vi "Kinesis-Teste-Vector-3.vi"() -> ()   [LabVIEW 2014]
doc: "André Romero - 2017\nandretec@ifsc.usp.br"
uses:
  Basic-VIs/motorsGlobalVar.vi
  <vilib>/Instr/_visa.llb/VISA Configure Serial Port (Instr).vi
  C:/user-Lab/AndreTec/GITs/andretec/Thorlabs-Vector-Move/kinesisTec/Kinesis/Thorlabs.MotionControl.Controls.dll
  kinesisTec/Kinesis/Thorlabs.MotionControl.Controls.dll
panel:
  out "IsMoving Y":bool
  out "IsMoving X":bool
  out "Y":dbl[](array[numeric])
  out "X":dbl[](array[numeric])
  out "XY Graph 2":cluster{dbl[], dbl[]}(graph)={[0.0, 0.8660254037844387, -0.8660254037844384, 0.0], [1.0, -0.4999999999999998, -0.5000000000000004, 1.0]}
  in  "Adjust Motors":bool
  out "Process time":string="0:00:50"
  out "Progress %":dbl(slide) scale=0.0..100.0
  out "XY Graph":cluster{"Graph X":dbl[], "Graph Y":dbl[]}(graph)
  in  "Swap XY":bool
  out "stop cronometro":bool=TRUE
  in  "Stop Button":bool
  in  "Graph Y":dbl[](array[numeric])=[0.0, 0.0, 6.6674440298507465, 6.6674440298507465, 6.6674440298507465, 6.6674440298507465, 6.6674440298507465, 6.6674440298507465, 6.6674440298507465, 6.6674440298507465, 6.6674440298507465, 6.6674440298507465, 6.6674440298507465, 6.6674440298507465, 6.6674440298507465, 6.6674440298507465, 6.6674440298507465, 6.6674440298507465, 6.6674440298507465, 6.6674440298507465, 6.6674440298507465, 6.6674440298507465, 6.6674440298507465, 6.6674440298507465, 6.6674440298507465, 6.6674440298507465, 6.6674440298507465, 6.6674440298507465, 6.6674440298507465, 6.6674440298507465, 6.6674440298507465, 6.6674440298507465, 6.6674440298507465, 6.6674440298507465, 6.6674440298507465, 6.6674440298507465, 6.6674440298507465, 6.6674440298507465, 6.6674440298507465, 6.6674440298507465, 6.6674440298507465, 6.6674440298507465, 6.6674440298507465, 6.673128498134329, 6.673128498134329, 6.673128498134329, 6.673128498134329, 6.673128498134329, 6.687354244402985, 6.687354244402985, 6.687354244402985, 6.687354244402985, 6.687354244402985, 6.692543143656716, 6.692543143656716, 6.692543143656716, 6.692543143656716, 6.692543143656716, 6.692543143656716, 6.692543143656716, 6.692543143656716, 6.692543143656716, 6.692543143656716, 6.692543143656716, 6.692543143656716, 6.691522854477612, 6.691522854477612, 6.691522854477612, 6.691522854477612, 6.691522854477612, 6.680183069029851, 6.680183069029851, 6.680183069029851, 6.680183069029851, 6.680183069029851, 6.658640391791045, 6.658640391791045, 6.658640391791045, 6.658640391791045, 6.658640391791045, 6.644793610074627, 6.644793610074627, 6.644793610074627, 6.644793610074627, 6.644793610074627, 6.642490671641791, 6.642490671641791, 6.642490671641791, 6.642490671641791, 6.642490671641791, 6.642490671641791, 6.642490671641791, 6.642490671641791, 6.642490671641791, 6.642490671641791, 6.642490671641791, 6.642490671641791, 6.642490671641791, 6.642490671641791, 6.642490671641791, 6.647825326492537, 6.647825326492537, 6.647825326492537, 6.647825326492537, 6.647825326492537, 6.66543260261194, 6.66543260261194, 6.66543260261194, 6.66543260261194, 6.66543260261194, 6.685226212686567, 6.685226212686567, 6.685226212686567, 6.685226212686567, 6.685226212686567, 6.692484841417911, 6.692484841417911, 6.692484841417911, 6.692484841417911, 6.692484841417911, 6.692543143656716, 6.692543143656716, 6.692543143656716, 6.692543143656716, 6.692543143656716, 6.692543143656716, 6.692543143656716, 6.691464552238806, 6.691464552238806, 6.691464552238806, 6.691464552238806, 6.691464552238806, 6.679833255597015, 6.679833255597015, 6.679833255597015, 6.679833255597015, 6.679833255597015, 6.658057369402985, 6.658057369402985, 6.658057369402985, 6.658057369402985, 6.658057369402985, 6.644647854477612, 6.644647854477612, 6.644647854477612, 6.644647854477612, 6.644647854477612, 6.642548973880597, 6.642548973880597, 6.642548973880597, 6.642548973880597, 6.642548973880597, 6.642519822761194, 6.642519822761194, 6.642519822761194, 6.642519822761194, 6.642519822761194, 6.642519822761194, 6.642519822761194, 6.642519822761194, 6.643569263059701, 6.643569263059701, 6.643569263059701, 6.643569263059701, 6.643569263059701, 6.655521222014926, 6.655521222014926, 6.655521222014926, 6.655521222014926, 6.655521222014926, 6.677180503731344, 6.677180503731344, 6.677180503731344, 6.677180503731344, 6.677180503731344, 6.690531716417911, 6.690531716417911, 6.690531716417911, 6.690531716417911, 6.690531716417911, 6.692572294776119, 6.692572294776119, 6.692572294776119, 6.692572294776119, 6.692572294776119, 6.692572294776119, 6.692572294776119, 6.692572294776119, 6.692572294776119, 6.692572294776119, 6.692572294776119, 6.692572294776119, 6.691522854477612, 6.691522854477612, 6.691522854477612, 6.691522854477612, 6.691522854477612, 6.680008162313433, 6.680008162313433, 6.680008162313433, 6.680008162313433, 6.680008162313433, 6.668668376865671, 6.668668376865671, 6.668668376865671, 6.668668376865671, 6.668668376865671, 6.667502332089552, 6.667502332089552, 6.667502332089552, 6.667502332089552, 6.667502332089552, 6.667502332089552, 6.667502332089552, 6.667502332089552, 6.667502332089552, 6.667502332089552, 6.667502332089552, 6.667502332089552, 6.667531483208955, 6.667531483208955, 6.667531483208955, 6.667531483208955, 6.667531483208955, 6.667531483208955, 6.667531483208955, 6.667531483208955, 6.667531483208955, 6.667531483208955, 6.667531483208955, 6.667531483208955, 6.667531483208955, 6.667531483208955, 6.667531483208955, 6.667531483208955, 6.667531483208955, 6.667531483208955, 6.667531483208955, 6.667531483208955, 6.667531483208955, 6.667531483208955, 6.667531483208955, 6.667531483208955, 6.667531483208955, 6.667531483208955, 6.667531483208955, 6.667531483208955, 6.667531483208955, 6.667531483208955, 6.667531483208955, 6.667531483208955, 6.667531483208955, 6.667531483208955, 6.667531483208955, 6.667531483208955, 6.667531483208955, 6.6663945895522385, 6.6663945895522385, 6.6663945895522385, 6.6663945895522385, 6.6663945895522385, 6.662051072761194, 6.662051072761194, 6.662051072761194, 6.662051072761194, 6.662051072761194, 6.644035680970149, 6.644035680970149, 6.644035680970149, 6.644035680970149, 6.644035680970149, 6.606430736940299, 6.606430736940299, 6.606430736940299, 6.606430736940299, 6.606430736940299, 6.593924906716418, 6.593924906716418, 6.593924906716418, 6.593924906716418, 6.593924906716418, 6.574539412313433, 6.574539412313433, 6.574539412313433, 6.574539412313433, 6.574539412313433, 6.567484841417911, 6.567484841417911, 6.567484841417911, 6.567484841417911, 6.567484841417911, 6.567484841417911, 6.567484841417911, 6.567484841417911, 6.567484841417911, 6.567484841417911, 6.567484841417911, 6.567513992537314, 6.567513992537314, 6.567513992537314, 6.567513992537314, 6.567513992537314, 6.567513992537314, 6.567513992537314, 6.567513992537314, 6.567513992537314, 6.567513992537314, 6.567543143656716, 6.567543143656716, 6.567543143656716, 6.567543143656716, 6.567543143656716, 6.567543143656716, 6.567543143656716, 6.567543143656716, 6.567543143656716, 6.567543143656716, 6.567543143656716, 6.567543143656716, 6.567543143656716, 6.567543143656716, 6.567543143656716, 6.567543143656716, 6.567543143656716, 6.567543143656716, 6.567543143656716, 6.567543143656716, 6.567543143656716, 6.567543143656716, 6.567543143656716, 6.567543143656716, 6.567543143656716, 6.567543143656716, 6.567543143656716, 6.567543143656716, 6.567543143656716, 6.567543143656716, 6.567543143656716, 6.567543143656716, 6.567543143656716, 6.567543143656716, 6.567543143656716, 6.567543143656716, 6.567543143656716, 6.567543143656716, 6.567543143656716, 6.567543143656716, 6.567543143656716, 6.567543143656716, 6.567543143656716, 6.567543143656716, 6.567543143656716, 6.567543143656716, 6.567543143656716, 6.567543143656716, 6.567543143656716, 6.567543143656716, 6.567543143656716, 6.567543143656716, 6.567543143656716, 6.567543143656716, 6.5667852145522385, 6.5667852145522385, 6.5667852145522385, 6.5667852145522385, 6.5667852145522385, 6.555299673507463, 6.555299673507463, 6.555299673507463, 6.555299673507463, 6.555299673507463, 6.533523787313433, 6.533523787313433, 6.533523787313433, 6.533523787313433, 6.533523787313433, 6.525186567164179, 6.525186567164179, 6.525186567164179, 6.525186567164179, 6.525186567164179, 6.517490671641791, 6.517490671641791, 6.517490671641791, 6.517490671641791, 6.517490671641791, 6.517490671641791, 6.517490671641791, 6.517490671641791, 6.517490671641791, 6.517490671641791, 6.517519822761194, 6.517519822761194, 6.517519822761194, 6.517519822761194, 6.517519822761194, 6.517519822761194, 6.517519822761194, 6.517519822761194, 6.517519822761194, 6.517519822761194, 6.517548973880597, 6.517548973880597, 6.517548973880597, 6.517548973880597, 6.517548973880597, 6.517548973880597, 6.517548973880597, 6.517548973880597, 6.517548973880597, 6.517548973880597, 6.517548973880597, 6.517548973880597, 6.517548973880597, 6.517548973880597, 6.517548973880597, 6.517548973880597, 6.517548973880597, 6.517548973880597, 6.517548973880597, 6.517548973880597, 6.517548973880597, 6.517548973880597, 6.517548973880597, 6.517548973880597, 6.517548973880597, 6.517548973880597, 6.517548973880597, 6.517548973880597, 6.517548973880597, 6.517548973880597, 6.517548973880597, 6.517548973880597, 6.517548973880597, 6.517548973880597, 6.517548973880597, 6.517548973880597, 6.517548973880597, 6.517548973880597, 6.517548973880597, 6.517548973880597, 6.517548973880597, 6.517548973880597, 6.517548973880597, 6.517548973880597, 6.517548973880597, 6.517548973880597, 6.517548973880597, 6.517548973880597, 6.517548973880597, 6.517548973880597, 6.517548973880597, 6.517548973880597, 6.517548973880597, 6.517548973880597, 6.517548973880597, 6.517548973880597, 6.517548973880597, 6.517548973880597, 6.517548973880597, 6.517548973880597, 6.516674440298507, 6.516674440298507, 6.516674440298507, 6.516674440298507, 6.516674440298507, 6.504897388059701, 6.504897388059701, 6.504897388059701, 6.504897388059701, 6.504897388059701, 6.481926305970149, 6.481926305970149, 6.481926305970149, 6.481926305970149, 6.481926305970149, 6.456943796641791, 6.456943796641791, 6.456943796641791, 6.456943796641791, 6.456943796641791, 6.4330690298507465, 6.4330690298507465, 6.4330690298507465, 6.4330690298507465, 6.4330690298507465, 6.419717817164179, 6.419717817164179, 6.419717817164179, 6.419717817164179, 6.419717817164179, 6.417473180970149, 6.417473180970149, 6.417473180970149, 6.417473180970149, 6.417473180970149, 6.417473180970149]
  in  "Graph X":dbl[](array[numeric])=[0.0, 0.0, 3.605935167910448, 3.605935167910448, 3.605935167910448, 3.605935167910448, 3.605935167910448, 3.609987173507463, 3.609987173507463, 3.609987173507463, 3.609987173507463, 3.609987173507463, 3.627157182835821, 3.627157182835821, 3.627157182835821, 3.627157182835821, 3.627157182835821, 3.6520813899253732, 3.6520813899253732, 3.6520813899253732, 3.6520813899253732, 3.6520813899253732, 3.6770930503731343, 3.6770930503731343, 3.6770930503731343, 3.6770930503731343, 3.6770930503731343, 3.697323927238806, 3.697323927238806, 3.697323927238806, 3.697323927238806, 3.697323927238806, 3.705311333955224, 3.705311333955224, 3.705311333955224, 3.705311333955224, 3.705311333955224, 3.705311333955224, 3.705311333955224, 3.705311333955224, 3.705311333955224, 3.705311333955224, 3.705311333955224, 3.7063024720149254, 3.7063024720149254, 3.7063024720149254, 3.7063024720149254, 3.7063024720149254, 3.7175839552238807, 3.7175839552238807, 3.7175839552238807, 3.7175839552238807, 3.7175839552238807, 3.7291861007462686, 3.7291861007462686, 3.7291861007462686, 3.7291861007462686, 3.7291861007462686, 3.7303521455223883, 3.7303521455223883, 3.7303521455223883, 3.7303521455223883, 3.7303521455223883, 3.7303521455223883, 3.7303521455223883, 3.7303521455223883, 3.7303521455223883, 3.7303521455223883, 3.7303521455223883, 3.7303521455223883, 3.7366779384328357, 3.7366779384328357, 3.7366779384328357, 3.7366779384328357, 3.7366779384328357, 3.7554221082089554, 3.7554221082089554, 3.7554221082089554, 3.7554221082089554, 3.7554221082089554, 3.774137126865672, 3.774137126865672, 3.774137126865672, 3.774137126865672, 3.774137126865672, 3.7803463152985075, 3.7803463152985075, 3.7803463152985075, 3.7803463152985075, 3.7803463152985075, 3.7803463152985075, 3.7803463152985075, 3.7803463152985075, 3.7803463152985075, 3.7803463152985075, 3.7803463152985075, 3.7803463152985075, 3.7803463152985075, 3.7803463152985075, 3.7803463152985075, 3.781803871268657, 3.781803871268657, 3.781803871268657, 3.781803871268657, 3.781803871268657, 3.7941930970149254, 3.7941930970149254, 3.7941930970149254, 3.7941930970149254, 3.7941930970149254, 3.816027285447761, 3.816027285447761, 3.816027285447761, 3.816027285447761, 3.816027285447761, 3.828678871268657, 3.828678871268657, 3.828678871268657, 3.828678871268657, 3.828678871268657, 3.8303404850746268, 3.8303404850746268, 3.8303404850746268, 3.8303404850746268, 3.8303404850746268, 3.8303404850746268, 3.8303404850746268, 3.8303404850746268, 3.8303404850746268, 3.8303404850746268, 3.8303404850746268, 3.8303404850746268, 3.8368703358208953, 3.8368703358208953, 3.8368703358208953, 3.8368703358208953, 3.8368703358208953, 3.8447994402985075, 3.8447994402985075, 3.8447994402985075, 3.8447994402985075, 3.8447994402985075, 3.866633628731343, 3.866633628731343, 3.866633628731343, 3.866633628731343, 3.866633628731343, 3.8803346548507465, 3.8803346548507465, 3.8803346548507465, 3.8803346548507465, 3.8803346548507465, 3.8803346548507465, 3.8803346548507465, 3.8803346548507465, 3.8803346548507465, 3.8803346548507465, 3.8803346548507465, 3.8803346548507465, 3.8803346548507465, 3.8803346548507465, 3.8803346548507465, 3.8803346548507465, 3.8803346548507465, 3.8803346548507465, 3.886631296641791, 3.886631296641791, 3.886631296641791, 3.886631296641791, 3.886631296641791, 3.9054046175373136, 3.9054046175373136, 3.9054046175373136, 3.9054046175373136, 3.9054046175373136, 3.92411963619403, 3.92411963619403, 3.92411963619403, 3.92411963619403, 3.92411963619403, 3.9303288246268657, 3.9303288246268657, 3.9303288246268657, 3.9303288246268657, 3.9303288246268657, 3.9303288246268657, 3.9303288246268657, 3.9303288246268657, 3.9303288246268657, 3.9303288246268657, 3.9303288246268657, 3.9303288246268657, 3.9303288246268657, 3.9303288246268657, 3.9303288246268657, 3.9303288246268657, 3.9303288246268657, 3.936800373134328, 3.936800373134328, 3.936800373134328, 3.936800373134328, 3.936800373134328, 3.9445545708955225, 3.9445545708955225, 3.9445545708955225, 3.9445545708955225, 3.9445545708955225, 3.95536963619403, 3.95536963619403, 3.95536963619403, 3.95536963619403, 3.95536963619403, 3.95536963619403, 3.95536963619403, 3.95536963619403, 3.95536963619403, 3.95536963619403, 3.95536963619403, 3.95536963619403, 3.956652285447761, 3.956652285447761, 3.956652285447761, 3.956652285447761, 3.956652285447761, 3.961141557835821, 3.961141557835821, 3.961141557835821, 3.961141557835821, 3.961141557835821, 3.9795067630597014, 3.9795067630597014, 3.9795067630597014, 3.9795067630597014, 3.9795067630597014, 4.004518423507463, 4.004518423507463, 4.004518423507463, 4.004518423507463, 4.004518423507463, 4.0406366604477615, 4.0406366604477615, 4.0406366604477615, 4.0406366604477615, 4.0406366604477615, 4.048624067164179, 4.048624067164179, 4.048624067164179, 4.048624067164179, 4.048624067164179, 4.0553579757462686, 4.0553579757462686, 4.0553579757462686, 4.0553579757462686, 4.0553579757462686, 4.0553579757462686, 4.0553579757462686, 4.055387126865671, 4.055387126865671, 4.055387126865671, 4.055387126865671, 4.055387126865671, 4.055387126865671, 4.055387126865671, 4.055387126865671, 4.055387126865671, 4.055387126865671, 4.0553579757462686, 4.0553579757462686, 4.0553579757462686, 4.0553579757462686, 4.0553579757462686, 4.0553579757462686, 4.0553579757462686, 4.0553579757462686, 4.0553579757462686, 4.0553579757462686, 4.0553579757462686, 4.0553579757462686, 4.0553579757462686, 4.0553579757462686, 4.0553579757462686, 4.0553579757462686, 4.0553579757462686, 4.0553579757462686, 4.0553579757462686, 4.0553579757462686, 4.0553579757462686, 4.0553579757462686, 4.0553579757462686, 4.0553579757462686, 4.0553579757462686, 4.0553579757462686, 4.0553579757462686, 4.0553579757462686, 4.0553579757462686, 4.0553579757462686, 4.0553579757462686, 4.061800373134329, 4.061800373134329, 4.061800373134329, 4.061800373134329, 4.061800373134329, 4.06972947761194, 4.06972947761194, 4.06972947761194, 4.06972947761194, 4.06972947761194, 4.091534514925373, 4.091534514925373, 4.091534514925373, 4.091534514925373, 4.091534514925373, 4.105352145522388, 4.105352145522388, 4.105352145522388, 4.105352145522388, 4.105352145522388, 4.105381296641791, 4.105381296641791, 4.105381296641791, 4.105381296641791, 4.105381296641791, 4.105381296641791, 4.105381296641791, 4.1050897854477615, 4.1050897854477615, 4.1050897854477615, 4.1050897854477615, 4.1050897854477615, 4.0951784048507465, 4.0951784048507465, 4.0951784048507465, 4.0951784048507465, 4.0951784048507465, 4.073489972014926, 4.073489972014926, 4.073489972014926, 4.073489972014926, 4.073489972014926, 4.060954990671642, 4.060954990671642, 4.060954990671642, 4.060954990671642, 4.060954990671642, 4.023874766791045, 4.023874766791045, 4.023874766791045, 4.023874766791045, 4.023874766791045, 4.008687033582089, 4.008687033582089, 4.008687033582089, 4.008687033582089, 4.008687033582089, 4.005363805970149, 4.005363805970149, 4.005363805970149, 4.005363805970149, 4.005363805970149, 4.005363805970149, 4.005363805970149, 4.005363805970149, 4.005363805970149, 4.005363805970149, 4.005363805970149, 4.005363805970149, 4.005363805970149, 4.005363805970149, 4.005363805970149, 4.005363805970149, 4.005363805970149, 4.005392957089552, 4.005392957089552, 4.005392957089552, 4.005392957089552, 4.005392957089552, 4.005392957089552, 4.005392957089552, 4.005392957089552, 4.005392957089552, 4.005392957089552, 4.005392957089552, 4.005392957089552, 4.005392957089552, 4.005392957089552, 4.005392957089552, 4.005392957089552, 4.005392957089552, 4.005392957089552, 4.005392957089552, 4.005392957089552, 4.011631296641791, 4.011631296641791, 4.011631296641791, 4.011631296641791, 4.011631296641791, 4.019472947761194, 4.019472947761194, 4.019472947761194, 4.019472947761194, 4.019472947761194, 4.042852145522388, 4.042852145522388, 4.042852145522388, 4.042852145522388, 4.042852145522388, 4.080398787313433, 4.080398787313433, 4.080398787313433, 4.080398787313433, 4.080398787313433, 4.099113805970149, 4.099113805970149, 4.099113805970149, 4.099113805970149, 4.099113805970149, 4.103777985074627, 4.103777985074627, 4.103777985074627, 4.103777985074627, 4.103777985074627, 4.105410447761194, 4.105410447761194, 4.105410447761194, 4.105410447761194, 4.105410447761194, 4.105410447761194, 4.105410447761194, 4.105410447761194, 4.105381296641791, 4.105381296641791, 4.105381296641791, 4.105381296641791, 4.105381296641791, 4.098297574626866, 4.098297574626866, 4.098297574626866, 4.098297574626866, 4.098297574626866, 4.089989505597015, 4.089989505597015, 4.089989505597015, 4.089989505597015, 4.089989505597015, 4.06083838619403, 4.06083838619403, 4.06083838619403, 4.06083838619403, 4.06083838619403, 4.0553579757462686, 4.0553579757462686, 4.0553579757462686, 4.0553579757462686, 4.0553579757462686, 4.0553579757462686, 4.0553579757462686, 4.0553579757462686, 4.0553579757462686, 4.0553579757462686, 4.0553579757462686, 4.0553579757462686, 4.055387126865671, 4.055387126865671, 4.055387126865671, 4.055387126865671, 4.055387126865671, 4.055416277985074, 4.055416277985074, 4.055416277985074, 4.055416277985074, 4.055416277985074, 4.055416277985074, 4.055416277985074, 4.055416277985074, 4.055416277985074, 4.055416277985074, 4.055416277985074, 4.055416277985074, 4.055416277985074, 4.055416277985074, 4.055416277985074, 4.055416277985074, 4.055416277985074, 4.055416277985074, 4.055416277985074, 4.055416277985074, 4.055416277985074, 4.055416277985074, 4.055416277985074, 4.055416277985074, 4.055416277985074, 4.055416277985074, 4.055416277985074, 4.055416277985074, 4.055416277985074, 4.055416277985074, 4.055416277985074]
  out "GetPOS Y":dbl=6.417473180970149 format="%_6f"
  out "GetPOS X":dbl=4.055416277985074 format="%#_6f"
  out ".NET Refnum out 2":refnum<k24>
  out ".NET Refnum out 1":refnum<k24>
  out "Motor 2":bool
  out "Motor 1":bool
  in  "Acceleration (mm/s)":dbl=0.05
  in  "Iniciar":bool
  in  "Velocity (mm/s)":sgl=0.05
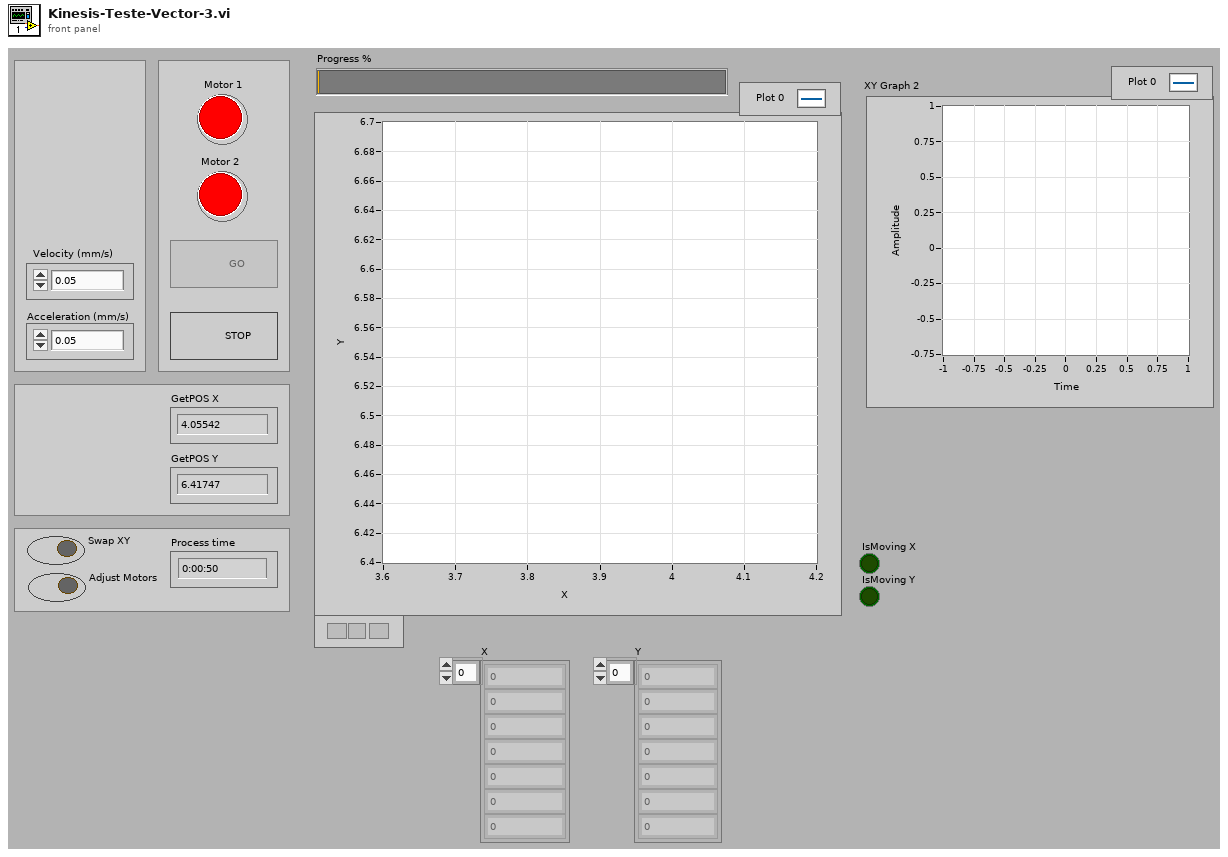
[diagram p1: front panel]
types:
  T1 = enum8{"Enabled", "Disabled", "Disabled and Grayed Out"}
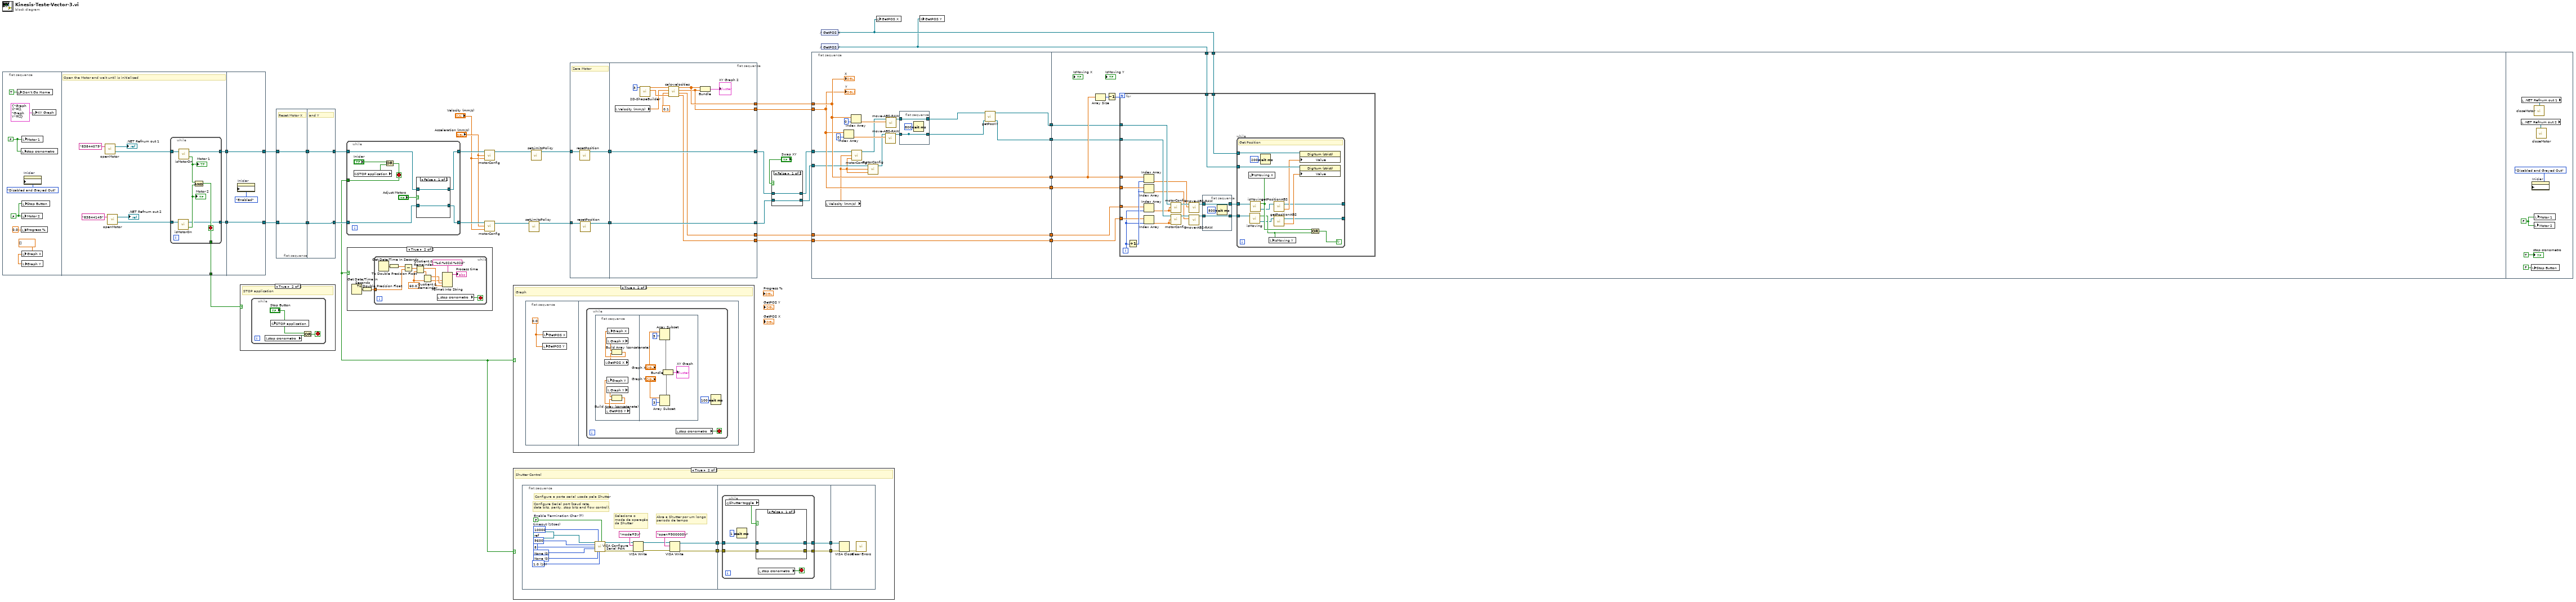
[diagram p0: block diagram]
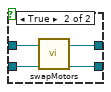
[diagram p2: hidden frame]
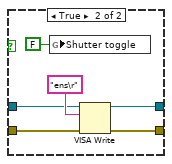
[diagram p4: hidden frame]
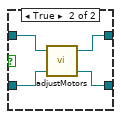
[diagram p8: hidden frame]
diagram:
  n1 = flat-sequence {
    tunnel: [w53] -> w27
    tunnel: [w52] -> w26
    tunnel: [w51] -> w25
    tunnel: [w62] -> w30
    tunnel: [w63] -> w31
    tunnel: w27 -> [w63]
    tunnel: w26 -> [w62]
    frame #0 {
      w40 = dbl[] [] ("Graph Y")
      w43 = FALSE ("Motor3\nLigado")
      w44 = FALSE
      n2 = global write "motorsGlobalVar.vi" "Don't Go Home"(TRUE ("Don't Go Home")) -> ()
      n3 = local write "stop cronometro"(w44) -> ()
      n4 = local write "Progress %"(0.0 ("Progress %")) -> ()
      n5 = local write "Motor 2"(w43) -> ()
      n6 = local write "Graph X"(w40) -> ()
      n7 = local write "Motor 1"(w44) -> ()
      n8 = local write "Stop Button"(w43) -> ()
      n9 = local write "Graph Y"(w40) -> ()
      n10 = property on="Iniciar" class="Bool (strict)"("DisabledEnum"=T1."Disabled and Grayed Out" ("Disabled")) -> ()  [unwired: 2 in, 2 out]
      n11 = local write "XY Graph"(cluster{"Graph X":dbl[], "Graph Y":dbl[]} {"Graph X"=[], "Graph Y"=[]} ("XY Graph")) -> ()
    }
    frame #1 {
      # "Open the Motor and wait until is initialized"
      n12 = call "openMotor.vi"("S/N Motor"="83844079") -> ("Device"=w49:refnum<k24>, ".NET Refnum out"=→".NET Refnum out 1":refnum<k24>)  [unwired: 1 in]
      n13 = call "openMotor.vi"("S/N Motor"="83844149") -> ("Device"=w50:refnum<k24>, ".NET Refnum out"=→".NET Refnum out 2":refnum<k24>)  [unwired: 1 in]
      n14 = while {
        tunnel: w49 -> [w58]
        tunnel: w50 -> [w57]
        tunnel: [w55] -> w53
        tunnel: [w54] -> w52
        tunnel: [w56] -> w51
        stop <- w56 stop-if-true
        n15 = call "isMotorOn.vi"("Device"=w57) -> ("isConnected"=w59:bool, "Device out"=w54:refnum<k24>)  [unwired: 1 in]
        "Motor 2" <- w59
        n16 = call "isMotorOn.vi"("Device"=w58) -> ("isConnected"=w60:bool, "Device out"=w55:refnum<k24>)  [unwired: 1 in]
        "Motor 1" <- w60
        n17 = And(x=w60, y=w59) -> (x .and. y?=w56:bool)
      }
    }
    frame #2 {
      n18 = property on="Iniciar" class="Bool (strict)"("DisabledEnum"=T1."Enabled" ("Disabled")) -> ()  [unwired: 2 in, 2 out]
    }
  }
  n19 = case shown="True" w25 {
    frame False {
    }
    frame True {
      # "STOP application"
      n20 = while {
        stop <- w65 stop-if-true
        n21 = local read "stop cronometro"() -> (w64:bool)
        n22 = global write "motorsGlobalVar.vi" "STOP application"("Stop Button") -> ()
        n23 = Or(x="Stop Button", y=w64) -> (x .or. y?=w65:bool)
      }
    }
  }
  n24 = flat-sequence {
    tunnel: w31 -> [w67]
    tunnel: w30 -> [w68]
    tunnel: [w67] -> w29
    tunnel: [w68] -> w28
    tunnel: [w70] -> w33
    tunnel: [w69] -> w32
    tunnel: w29 -> [w70]
    tunnel: w28 -> [w69]
    frame #0 {
      # "Reset Motor X"
    }
    frame #1 {
      # "and Y"
    }
  }
  n25 = while {
    tunnel: [w78] -> w24
    tunnel: w33 -> [w73]
    tunnel: w32 -> [w74]
    tunnel: [w72] -> w37
    tunnel: [w71] -> w36
    stop <- w78 stop-if-true
    n26 = global read "motorsGlobalVar.vi" "STOP application"() -> (w76:bool)
    n27 = Or(x="Iniciar", y=w76) -> (x .or. y?=w78:bool)
    n28 = case shown="False" "Adjust Motors" {
      tunnel: w74 -> [w79 w84]
      tunnel: w73 -> [w80 w83]
      tunnel: [w80 w82] -> w72
      tunnel: [w79 w81] -> w71
      frame False {
      }
      frame True {
        n29 = call "adjustMotors.vi"("Device 2"=w84, "Device 1"=w83) -> ("Device out 2"=w81:refnum<k24>, "Device out 1"=w82:refnum<k24>)  [unwired: 2 in]
      }
    }
  }
  n30 = case shown="True" w24 {
    frame False {
    }
    frame True {
      n31 = Get Date/Time In Seconds() -> (seconds since 1Jan1904=w86:timestamp)
      n32 = To Double Precision Float(number=w86) -> (double precision float=w85:dbl)
      n33 = while {
        tunnel: w85 -> [w90]
        stop <- w98 stop-if-true
        w95 = 60.0 ("y")
        n34 = Get Date/Time In Seconds() -> (seconds since 1Jan1904=w97:timestamp)
        n35 = To Double Precision Float(number=w97) -> (double precision float=w91:dbl)
        n36 = Subtract(x=w91, y=w90) -> (x-y=w89:dbl)
        n37 = Quotient & Remainder(x=w89, y=w95) -> (x-y*floor(x/y)=w94:dbl, floor(x/y)=w96:dbl)
        n38 = Quotient & Remainder(x=w96, y=w95) -> (x-y*floor(x/y)=w93:dbl, floor(x/y)=w92:dbl)
        n39 = local read "stop cronometro"() -> (w98:bool)
        n40 = Format Into String(format string="%d:%02d:%02d", w92, w93, w94) -> (resulting string=→"Process time":string)  [unwired: 2 in, 1 out]
      }
    }
  }
  n41 = call "motorConfig.vi"("Velocity"="Velocity (mm/s)", "Acceleration"="Acceleration (mm/s)", "Device in"=w37) -> ("Device out"=w23:refnum<k24>)  [unwired: 2 in]
  n42 = call "motorConfig.vi"("Velocity"="Velocity (mm/s)", "Acceleration"="Acceleration (mm/s)", "Device in"=w36) -> ("Device out"=w21:refnum<k24>)  [unwired: 2 in]
  n43 = case shown="True" w24 {
    frame False {
    }
    frame True {
      # "Graph"
      n44 = flat-sequence {
        frame #0 {
          w99 = 0.0
          n45 = local write "GetPOS Y"(w99) -> ()
          n46 = local write "GetPOS X"(w99) -> ()
        }
        frame #1 {
          n47 = while {
            stop <- w100 stop-if-true
            n48 = flat-sequence {
              frame #0 {
                n49 = local read "GetPOS X"() -> (w105:dbl)
                n50 = local read "GetPOS Y"() -> (w104:dbl)
                n51 = local read "Graph X"() -> (w107:dbl[])
                n52 = local read "Graph Y"() -> (w102:dbl[])
                n53 = Build Array (concatenate)(w107, w105) -> (w106:dbl[])
                n54 = local write "Graph X"(w106) -> ()
                n55 = Build Array (concatenate)(w102, w104) -> (w103:dbl[])
                n56 = local write "Graph Y"(w103) -> ()
              }
              frame #1 {
                n57 = Array Subset(array="Graph Y", index=3) -> (w108:dbl[])  [unwired: 1 in]
                n58 = Array Subset(array="Graph X", index=3) -> (w111:dbl[])  [unwired: 1 in]
                n59 = Bundle(w111, w108) -> (→"XY Graph":cluster{dbl[], dbl[]})  [unwired: 1 in]
              }
            }
            n60 = local read "stop cronometro"() -> (w100:bool)
            n61 = Wait (ms)(milliseconds to wait=u32 100) -> ()  [unwired: 1 out]
          }
        }
      }
    }
  }
  n62 = case shown="True" w24 {
    frame False {
    }
    frame True {
      # "Shutter Control"
      n63 = flat-sequence {
        tunnel: [w120] -> w118
        tunnel: [w119] -> w117
        tunnel: w118 -> [w138]
        tunnel: w117 -> [w135]
        tunnel: [w137] -> w116
        tunnel: [w136] -> w115
        tunnel: w116 -> [w156]
        tunnel: w115 -> [w155]
        frame #0 {
          w130 = u16 0 items=["None", "Odd", "Even", "Mark", "Space"] ("parity")
          w127 = u16 10 items=["1.0"=10, "1.5"=15, "2.0"=20] ("stop bits")
          w126 = u16 0 items=["None"=0, "XON/XOFF"=1, "RTS/CTS"=2, "DTR/DSR"=4] ("flow control")
          w128 = FALSE  # Enable Termination Char (T)
          w129 = u32 10000  # timeout (10sec)
          # "Configura a porta serial usada pela Shutter"
          # "Configure Serial port (baud rate,\ndata bits, parity, stop bits and flow control)."
          # "Seleciona o \nmode de operação\nda Shutter"
          # "Abre a Shutter por um longo\nperíodo de tempo"
          n64 = call-poly "VISA Configure Serial Port"("VISA resource name"=refnum<visa-resource-name> "COM3", "timeout (10sec)"=w129, "Enable Termination\nChar (T)"=w128, "baud rate (9600)"=u32 9600 ("baud rate"), "data bits (8)"=u16 8 ("data bits"), "parity (0:none)"=w130, "stop bits (10: 1 bit)"=w127, "flow control (0:none)"=w126) -> ("VISA resource name out"=w124:refnum<visa-resource-name>, "error out"=w123:errorcluster)  [unwired: 6 in]
          n65 = VISA Write(VISA resource name=w124, write buffer="mode=3\r", error in (no error)=w123) -> (VISA resource name out=w122:refnum<visa-resource-name>, error out=w121:errorcluster)  [unwired: 1 out]
          n66 = VISA Write(VISA resource name=w122, write buffer="open=900000\r", error in (no error)=w121) -> (VISA resource name out=w120:refnum<visa-resource-name>, error out=w119:errorcluster)  [unwired: 1 out]
        }
        frame #1 {
          n67 = while {
            tunnel: w138 -> [w145]
            tunnel: [w144] -> w137
            tunnel: [w143] -> w136
            tunnel: w135 -> [w142]
            stop <- w139 stop-if-true
            n68 = global read "motorsGlobalVar.vi" "Shutter toggle"() -> (w141:bool)
            n69 = Wait (ms)(milliseconds to wait=u32 1) -> ()  [unwired: 1 out]
            n70 = case shown="False" w141 {
              tunnel: w145 -> [w147 w152]
              tunnel: [w147 w151] -> w144
              tunnel: [w146 w150] -> w143
              tunnel: w142 -> [w146 w149]
              frame False {
              }
              frame True {
                n71 = global write "motorsGlobalVar.vi" "Shutter toggle"(FALSE ("Shutter toggle")) -> ()
                n72 = VISA Write(VISA resource name=w152, write buffer="ens\r", error in (no error)=w149) -> (VISA resource name out=w151:refnum<visa-resource-name>, error out=w150:errorcluster)  [unwired: 1 out]
              }
            }
            n73 = local read "stop cronometro"() -> (w139:bool)
          }
        }
        frame #2 {
          n74 = VISA Close(VISA resource name=w156, error in (no error)=w155) -> (error out=w154:errorcluster)
          n75 = call <vilib>:"Clear Errors.vi"("error in (no error)"=w154) -> ()  [unwired: 5 in, 2 out]
        }
      }
    }
  }
  n76 = call "setLimitsPolicy.vi"("Device in"=w21) -> ("Device out"=w20:refnum<k24>)  [unwired: 10 in]
  n77 = call "setLimitsPolicy.vi"("Device in"=w23) -> ("Device out"=w22:refnum<k24>)  [unwired: 10 in]
  n78 = flat-sequence {
    tunnel: w22 -> [w160]
    tunnel: w20 -> [w158]
    tunnel: [w159] -> w19
    tunnel: [w157] -> w18
    tunnel: [w171] -> w15
    tunnel: [w172] -> w16
    tunnel: w19 -> [w172]
    tunnel: w18 -> [w171]
    tunnel: [w164] -> w12
    tunnel: [w163] -> w11
    tunnel: [w162] -> w8
    tunnel: [w161] -> w7
    frame #0 {
      # "Zera Motor"
      n79 = call "resetPosition.vi"("Device in"=w160) -> ("Device out"=w159:refnum<k24>)  [unwired: 10 in]
      n80 = call "resetPosition.vi"("Device in"=w158) -> ("Device out"=w157:refnum<k24>)  [unwired: 10 in]
    }
    frame #1 {
      n81 = local read "Velocity (mm/s)"() -> (w167:sgl)
      n82 = call "2D-ShapeBuilder.vi"("Number of Sides"=3) -> ("Y out"=w168:dbl[], "X out"=w169:dbl[])  [unwired: 9 in]
      n83 = call "calc-velocities.vi"("Y in"=w168, "Radius"=0.1, "Velocidade (mm/s)"=w167, "X in"=w169) -> ("Vy"=w161:ext[], "Vx"=w162:ext[], "Y"=w163:dbl[], "X"=w164:dbl[])  [unwired: 2 in, 2 out]
      n84 = Bundle("X"=w164, "Y"=w163) -> (→"XY Graph 2":cluster{"X":dbl[], "Y":dbl[]})  [unwired: 1 in]
    }
  }
  n85 = case shown="False" "Swap XY" {
    tunnel: w16 -> [w174 w178]
    tunnel: w15 -> [w173 w177]
    tunnel: [w174 w176] -> w14
    tunnel: [w173 w175] -> w13
    frame False {
    }
    frame True {
      n86 = call "swapMotors.vi"("Device 2"=w177, "Device 1"=w178) -> ("Device out 1"=w175:refnum<k24>, "Device out 2"=w176:refnum<k24>)  [unwired: 2 in, 2 out]
    }
  }
  n87 = flat-sequence {
    tunnel: w13 -> [w190]
    tunnel: w14 -> [w191]
    tunnel: w12 -> [w193]
    tunnel: w11 -> [w192]
    tunnel: [w193] -> w10
    tunnel: [w192] -> w9
    tunnel: w8 -> [w187]
    tunnel: w7 -> [w186]
    tunnel: [w187] -> w6
    tunnel: [w186] -> w5
    tunnel: [w185] -> w4
    tunnel: [w181] -> w3
    tunnel: w10 -> [w208]
    tunnel: w9 -> [w210]
    tunnel: w6 -> [w207]
    tunnel: w5 -> [w206]
    tunnel: w4 -> [w205]
    tunnel: w3 -> [w204]
    tunnel: w2 -> [w203]
    tunnel: w1 -> [w202]
    frame #0 {
      n88 = local read "Velocity (mm/s)"() -> (w182:sgl)
      n89 = Index Array(array=w192, index=0) -> (element=w195:dbl)
      n90 = Index Array(array=w193, index=0) -> (element=w194:dbl)
      n91 = call "motorConfig.vi"("Velocity"=w182, "Acceleration"=w182, "Device in"=w191) -> ("Device out"=w189:refnum<k24>)  [unwired: 2 in]
      n92 = call "motorConfig.vi"("Velocity"=w182, "Acceleration"=w182, "Device in"=w190) -> ("Device out"=w188:refnum<k24>)  [unwired: 2 in]
      n93 = call "move-ABS-RAW.vi"("position"=w195, "Device in"=w188) -> ("Device out"=w183:refnum<k24>)  [unwired: 9 in]
      n94 = call "move-ABS-RAW.vi"("position"=w194, "Device in"=w189) -> ("Device out"=w184:refnum<k24>)  [unwired: 9 in]
      n95 = flat-sequence {
        tunnel: w184 -> [w200]
        tunnel: [w200] -> w180
        tunnel: w183 -> [w198]
        tunnel: [w198] -> _
        tunnel: [w198] -> w179
        frame #0 {
          n96 = Wait (ms)(milliseconds to wait=u32 800) -> ()  [unwired: 1 out]
        }
      }
      n97 = call "getPosXY.vi"("Device Y in"=w179, "Device X in"=w180) -> ("Device Y out"=w181:refnum<k24>, "Device X out"=w185:refnum<k24>)  [unwired: 7 in, 1 out]
      "X" <- w193
      "Y" <- w192
    }
    frame #1 {
      n98 = Array Size(array=w208) -> (size(s)=w209:i32)
      n99 = Decrement(x=w209) -> (x-1=w201:i32)
      n100 = for {
        N: w201 -> [_]
        tunnel: w208 -> [w230]
        tunnel: w210 -> [w229]
        tunnel: w207 -> [w227]
        tunnel: w206 -> [w226]
        tunnel: w205 -> [w224]
        tunnel: w204 -> [w223]
        tunnel: w203 -> [w216]
        tunnel: w202 -> [w215]
        i -> [w225]
        n101 = Increment(x=w225) -> (x+1=w228:i32)
        n102 = Index Array(array=w230, index=w228) -> (element=w218:dbl)
        n103 = Index Array(array=w229, index=w228) -> (element=w217:dbl)
        n104 = Index Array(array=w227, index=w225) -> (element=w221:ext)
        n105 = Index Array(array=w226, index=w225) -> (element=w222:ext)
        n106 = call "motorConfig.vi"("Velocity"=w221, "Acceleration"=w221, "Device in"=w224) -> ("Device out"=w220:refnum<k24>)  [unwired: 2 in]
        n107 = call "motorConfig.vi"("Velocity"=w222, "Acceleration"=w222, "Device in"=w223) -> ("Device out"=w219:refnum<k24>)  [unwired: 2 in]
        n108 = call "move-ABS-RAW.vi"("position"=w218, "Device in"=w220) -> ("Device out"=w214:refnum<k24>)  [unwired: 9 in]
        n109 = call "move-ABS-RAW.vi"("position"=w217, "Device in"=w219) -> ("Device out"=w212:refnum<k24>)  [unwired: 9 in]
        n110 = flat-sequence {
          tunnel: w214 -> [w233]
          tunnel: [w233] -> w213
          tunnel: w212 -> [w232]
          tunnel: [w232] -> w211
          frame #0 {
            n111 = Wait (ms)(milliseconds to wait=u32 800) -> ()  [unwired: 1 out]
          }
        }
        n112 = while {
          tunnel: w213 -> [w238]
          tunnel: w216 -> [w247]
          tunnel: w215 -> [w246]
          tunnel: [w241] -> _
          tunnel: [w240] -> _
          tunnel: w211 -> [w239]
          stop <- w243 continue-if-true
          # "Get Position"
          n113 = call "isMoving.vi"("Device in"=w239) -> ("Device out"=w234:refnum<k24>, "IsMoving"=w236:bool)  [unwired: 1 in]
          n114 = call "isMoving.vi"("Device in"=w238) -> ("Device out"=w235:refnum<k24>, "IsMoving"=w237:bool)  [unwired: 1 in]
          n115 = local write "IsMoving X"(w237) -> ()
          n116 = Wait (ms)(milliseconds to wait=u32 200) -> ()  [unwired: 1 out]
          n117 = local write "IsMoving Y"(w236) -> ()
          n118 = call "getPositionABS.vi"("Device"=w235) -> ("GetPOS"=w245:dbl, "Device out"=w241:refnum<k24>)  [unwired: 1 in]
          n119 = call "getPositionABS.vi"("Device"=w234) -> ("GetPOS"=w244:dbl, "Device out"=w240:refnum<k24>)  [unwired: 1 in]
          n120 = property class="DigNum (strict)"(reference=w247, "Value"=w245) -> ()  [unwired: 1 in, 2 out]
          n121 = property class="DigNum (strict)"(reference=w246, "Value"=w244) -> ()  [unwired: 1 in, 2 out]
          n122 = Or(x=w237, y=w236) -> (x .or. y?=w243:bool)
        }
      }
    }
    frame #2 {
      w253 = FALSE
      n123 = local read ".NET Refnum out 2"() -> (w248:refnum<k24>)
      n124 = local read ".NET Refnum out 1"() -> (w249:refnum<k24>)
      n125 = local write "Stop Button"(FALSE ("Stop Button")) -> ()
      n126 = property on="Iniciar" class="Bool (strict)"("DisabledEnum"=T1."Disabled and Grayed Out" ("Disabled")) -> ()  [unwired: 2 in, 2 out]
      n127 = call "closeMotor.vi"(".NET Refnum in"=w249) -> ()  [unwired: 2 in]
      n128 = local write "Motor 2"(w253) -> ()
      n129 = local write "Motor 1"(w253) -> ()
      n130 = call "closeMotor.vi"(".NET Refnum in"=w248) -> ()  [unwired: 2 in]
      "stop cronometro" <- TRUE ("stop cronometro")
    }
  }
  n131 = control-ref of="GetPOS X"() -> (w2:refnum<vi>)
  n132 = control-ref of="GetPOS Y"() -> (w1:refnum<vi>)
  n133 = global write "motorsGlobalVar.vi" "GetPOS X"(w2) -> ()
  n134 = global write "motorsGlobalVar.vi" "GetPOS Y"(w1) -> ()
